vi "Send Message, JSON Payload.vi"(0 "IPEndPoint":T1, 7 "Message":string, 9 "Payload":string="{}", 11 "error in (no error)":errorcluster) -> (4 "IPEndPoint thru":T1, 15 "error out":errorcluster)   [LabVIEW 2020, in "epl-network.lvlib"]
uses:
  epl-network.lvlib
  Typedefs/IPEndPoint.ctl
  Typedefs/TCP Message.ctl
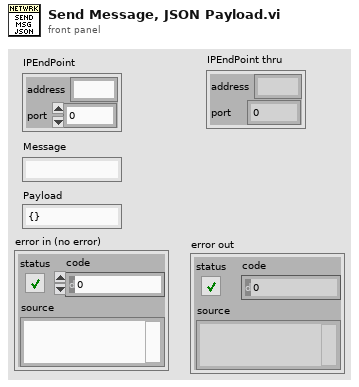
[diagram p1: front panel]
types:
  T1 = typedef "epl-network.lvlib/IPEndPoint.ctl" = cluster{"address":string, "port":i32}
  T2 = typedef "epl-network.lvlib/TCP Message.ctl" = cluster{"Code":i32, "Command":string, "Payload":string}
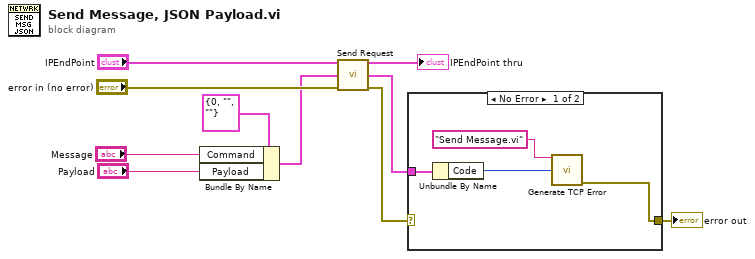
[diagram p0: block diagram]
diagram:
  n1 = Bundle By Name(cluster=T2 {"Code"=0, "Command"="", "Payload"=""} ("TCPMessage"), "Command"="Message", "Payload"="Payload") -> (w6:T2)
  n2 = call "Send Request.vi"("IPEndPoint"="IPEndPoint", "TCPMessage"=w6, "error in (no error)"="error in (no error)") -> ("IPEndPoint thru"=→"IPEndPoint thru":T1, "Response"=w3:T2, "error out"=w4:errorcluster)  [unwired: 10 in]
  n3 = case shown="No Error" w4 {
    selector: w4 -> [_ w15]
    tunnel: w3 -> [w14 _]
    tunnel: [w12 w15] -> w2
    frame No Error {
      n4 = Unbundle By Name(w14) -> ("Code"=w13:i32)
      n5 = call "Generate TCP Error.vi"("VI Name"="Send Message.vi", "TCP response code"=w13) -> ("error out"=w12:errorcluster)  [unwired: 13 in]
    }
    frame Error {
    }
  }
  "error out" <- w2
